vi "1_FindWorkingZDistance.vi"(0 "Inputs: Collect Images":T3={"Image feed"=refnum, "Axes Speeds [mm/s]"={"X Speed"=10.0, "Y Speed"=10.0, "Z Speed"=10.0}, "XYZ .NET Refnum in"=refnum, "Stage position"=refnum, "Moving"=refnum}, 1 "Current Build Phase":refnum<vi>, 2 "Autofocus Coordinates":T5, 3 "Focusing test range [mm]":dbl, 4 "Stepsize [mm]":dbl, 5 "error in (no error)":errorcluster, 6 "Templates directory":path, 8 "Path to save collected images":path=path "E:/XYZstage+Camera_CollectedImages/12-17-2016/images", 9 "milliseconds to wait":u32=3500) -> (14 "Optimized working distance":dbl, 15 "Uncertainty on optimized Z":dbl, 16 "Outputs: Collect Images":T1, 19 "error out":errorcluster)   [LabVIEW 2016]
uses:
  C:/Users/Aerotech/Documents/BNL_ThermomechanicalStave/AerotechLibraries/Bin/Aerotech.A3200.dll
  AerotechLibraries/Bin/Aerotech.A3200.dll
panel:
  out "Radius vs Height: Linear Fit Results":T4
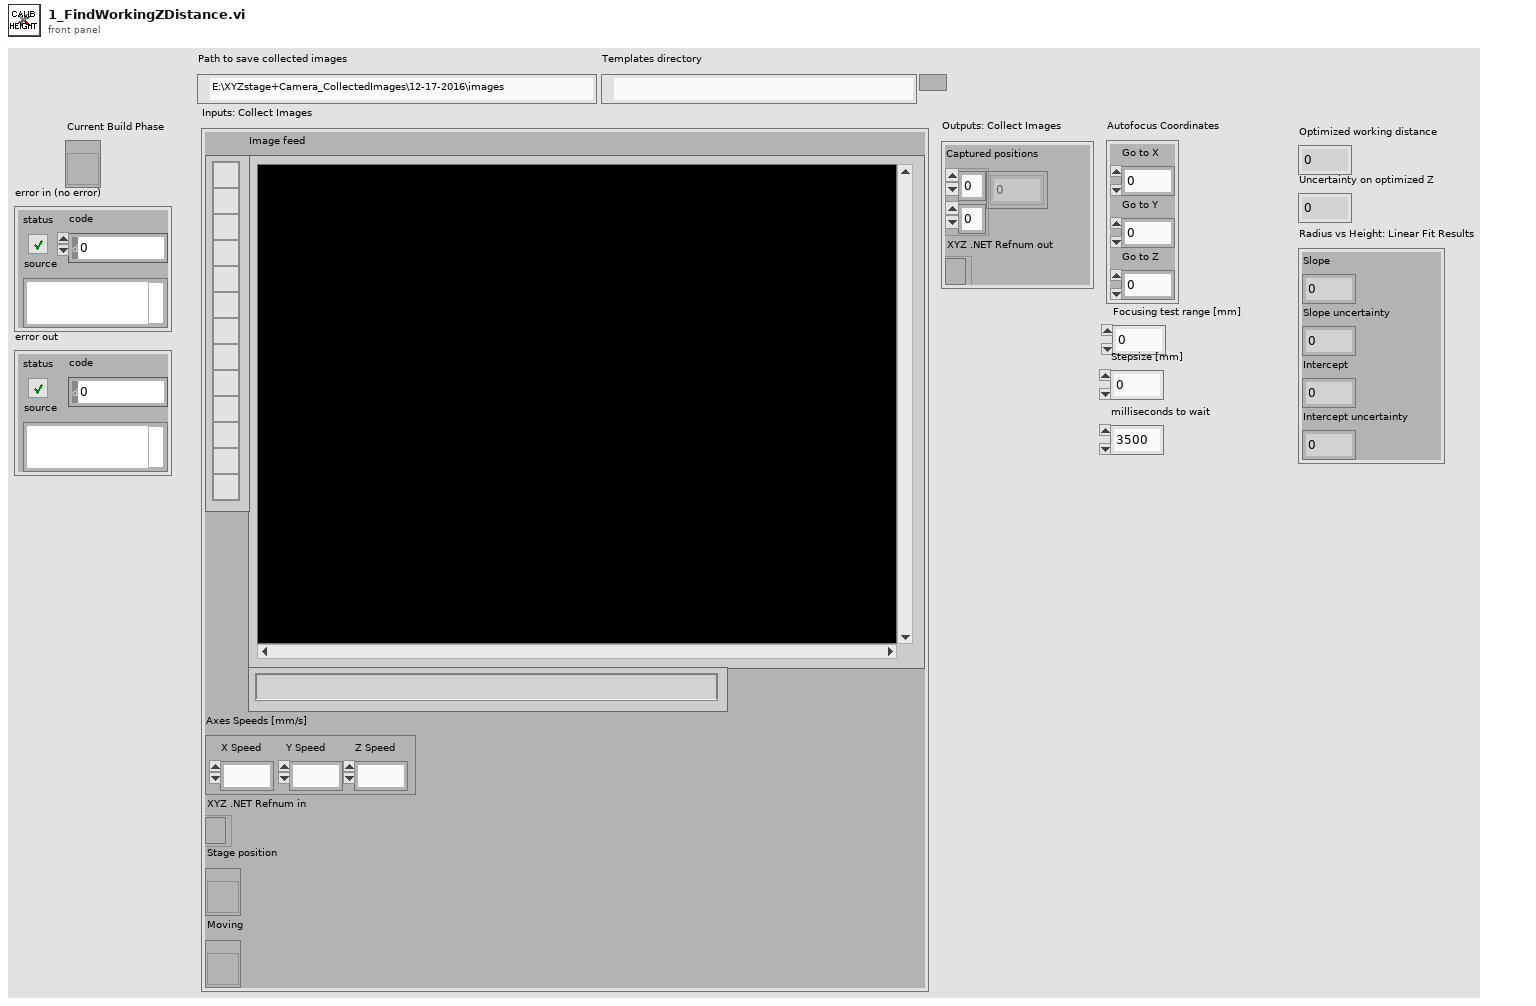
[diagram p1: front panel]
types:
  T1 = cluster{"Captured positions":dbl[][], "XYZ .NET Refnum out":refnum<k24>}
  T2 = typedef "IMAQ Image.ctl" = refnum<image>
  T3 = cluster{"Image feed":T2, "Axes Speeds [mm/s]":cluster{"X Speed":dbl, "Y Speed":dbl, "Z Speed":dbl}, "XYZ .NET Refnum in":refnum<k24>, "Stage position":refnum<vi>, "Moving":refnum<vi>}
  T4 = cluster{"Slope":dbl, "Slope uncertainty":dbl, "Intercept":dbl, "Intercept uncertainty":dbl}
  T5 = cluster{"Go to X":dbl, "Go to Y":dbl, "Go to Z":dbl}
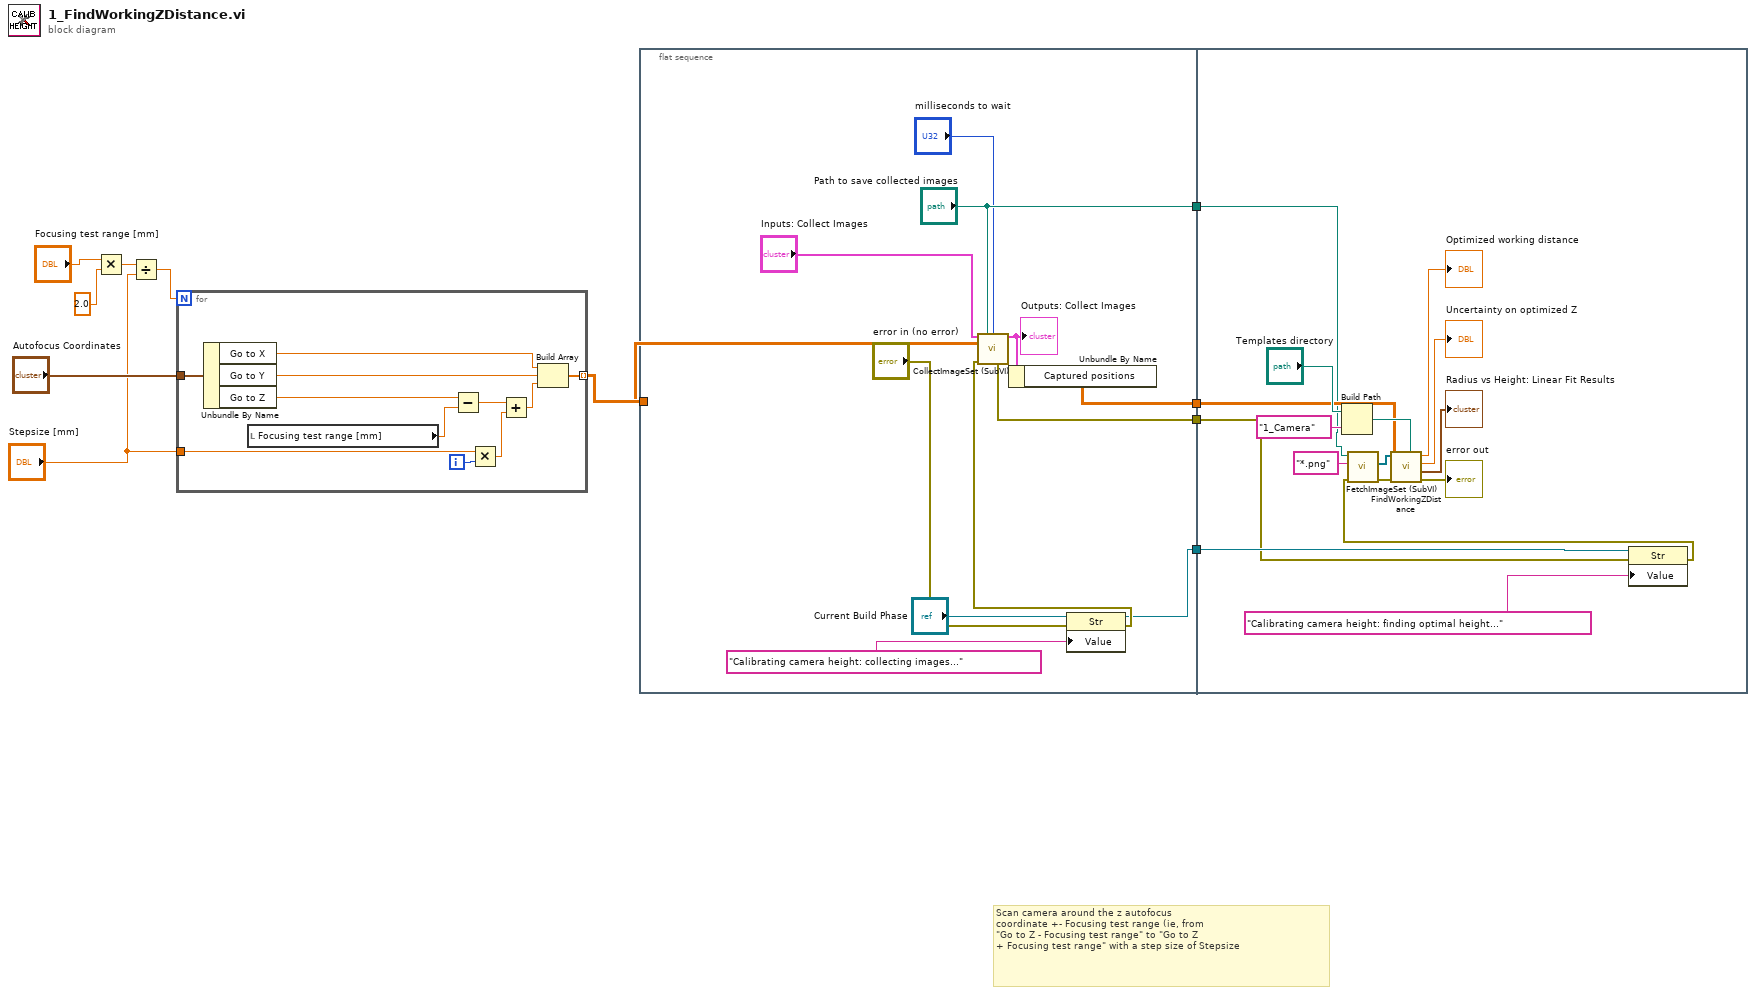
[diagram p0: block diagram]
diagram:
  # "Scan camera around the z autofocus\ncoordinate +- Focusing test range (ie, from\n\"Go to Z - Focusing test range\" to \"Go to Z \n+ Focusing test range\" with a step size of Stepsize"
  n1 = Multiply(x="Focusing test range [mm]", y=2.0) -> (x*y=w6:dbl)
  n2 = Divide(x=w6, y="Stepsize [mm]") -> (x/y=w8:dbl)
  n3 = for {
    N: w8 -> [_]
    tunnel: "Autofocus Coordinates" -> [w22]
    tunnel: [w19] -> w10 mode=indexing
    tunnel: "Stepsize [mm]" -> [w17]
    i -> [w18]
    n4 = Unbundle By Name(w22) -> ("Go to X"=w21:dbl, "Go to Y"=w20:dbl, "Go to Z"=w16:dbl)
    n5 = local read "Focusing test range [mm]"() -> (w15:dbl)
    n6 = Subtract(x=w16, y=w15) -> (x-y=w14:dbl)
    n7 = Multiply(x=w17, y=w18) -> (x*y=w13:dbl)
    n8 = Add(x=w14, y=w13) -> (x+y=w12:dbl)
    n9 = Build Array(w21, w20, w12) -> (w19:dbl[])
  }
  n10 = flat-sequence {
    tunnel: w10 -> [w31]
    tunnel: [w26] -> w4
    tunnel: [w32] -> w3
    tunnel: ["Path to save collected images"] -> w2
    tunnel: [w23] -> w1
    tunnel: w4 -> [w36]
    tunnel: w3 -> [w42]
    tunnel: w2 -> [w38]
    tunnel: w1 -> [w37]
    frame #0 {
      n11 = property class="Str"(reference="Current Build Phase", error in="error in (no error)", "Value"="Calibrating camera height: collecting images...") -> (reference out=w23:refnum<vi>, error out=w24:errorcluster)
      n12 = call "CollectImageSet (SubVI).vi"("Inputs"="Inputs: Collect Images", "Path to save collected images"="Path to save collected images", "milliseconds to wait"="milliseconds to wait", "Set of coordinates to process"=w31, "error in"=w24) -> ("Outputs"=w27:T1, "error out"=w26:errorcluster)  [unwired: 8 in, 1 out]
      "Outputs: Collect Images" <- w27
      n13 = Unbundle By Name(w27) -> ("Captured positions"=w32:dbl[][])
    }
    frame #1 {
      n14 = Build Path(base path="Templates directory", name or relative path="1_Camera") -> (appended path=w43:path)
      n15 = property class="Str"(reference=w37, error in=w36, "Value"="Calibrating camera height: finding optimal height...") -> (error out=w35:errorcluster)  [unwired: 1 out]
      n16 = call "FetchImageSet (SubVI).vi"("error in (no error)"=w35, "Naming Convention"="*.png", "Images Directory"=w38) -> ("error out"=w39:errorcluster, "Image Array"=w41:T2[])  [unwired: 6 in, 1 out]
      n17 = call "FindWorkingZDistance.vi"("Template File Path"=w43, "error in"=w39, "Capture coordinates"=w42, "Images Array"=w41) -> ("error out"=→"error out":errorcluster, "Radius vs Height: Linear Fit Results"=→"Radius vs Height: Linear Fit Results":T4, "Uncertainty on optimized Z"=→"Uncertainty on optimized Z":dbl, "Optimized Z"=→"Optimized working distance":dbl)  [unwired: 4 in]
    }
  }
